vi "update facade.vi"(0 "control ref":refnum<vi>, 2 "Data In":T1, 4 "index":i32) -> (19 "error out":errorcluster)   [LabVIEW 2014, in "X DIM conditions.xctl"]
uses:
  X DIM conditions.xctl
  X DIM conditions.Data.ctl
  PTSequencer/PTSequencer.DIM service condition.ctl
  CS_Core/CSSystem/CoreDefs/CoreDefs.rawDataType.ctl
  PTSequencer/PTSequencer.lvlib
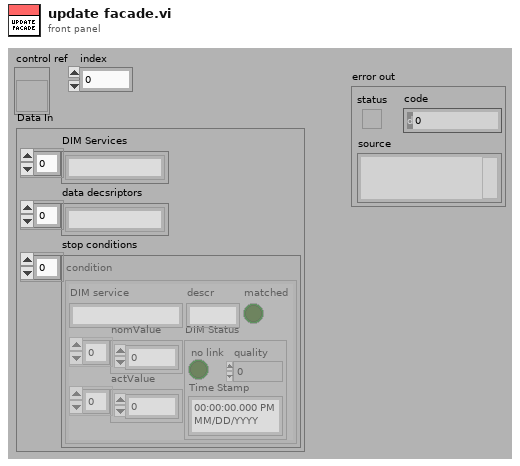
[diagram p1: front panel]
types:
  T1 = typedef "X DIM conditions.xctl/X DIM conditions.Data.ctl" = cluster{"DIM Services":string[], "data decsriptors":string[], "stop conditions":T2[]}
  T2 = typedef "PTSequencer.lvlib/PTSequencer.DIM service condition.ctl" = cluster{"DIM service":string, "descr":string, "nomValue":T3, "actValue":T3, "matched":bool, "DIM Status":cluster{"no link":bool, "quality":i32, "Time Stamp":timestamp}}
  T3 = typedef "CoreDefs.rawDataType.ctl" = i8[]
  T4 = enum8{"Enabled", "Disabled", "Disabled and Grayed Out"}
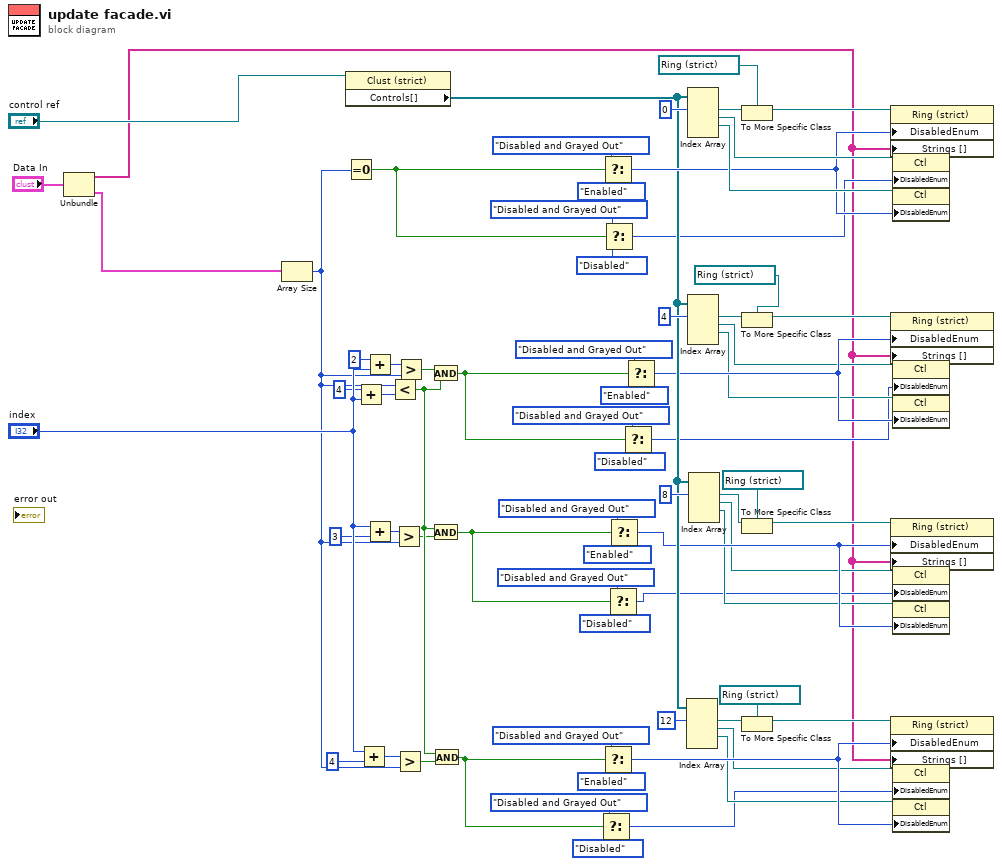
[diagram p0: block diagram]
diagram:
  n1 = Unbundle("Data In") -> ("DIM Services"=w1:string[], "stop conditions"=w69:T2[])  [unwired: 1 out]
  n2 = Array Size(array=w69) -> (size(s)=w43:i32)
  n3 = property class="Clust (strict)"(reference="control ref") -> ("Controls[]"=w39:refnum<vi>[])  [unwired: 1 in, 2 out]
  n4 = Equal To 0?(x=w43) -> (x = 0?=w6:bool)
  n5 = Add(x=4, y="index") -> (x+y=w52:i32)
  n6 = Add(x="index", y=4) -> (x+y=w56:i32)
  n7 = Add(x=2, y="index") -> (x+y=w53:i32)
  n8 = Add(x="index", y=3) -> (x+y=w55:i32)
  n9 = Less?(x=w43, y=w52) -> (x < y?=w50:bool)
  n10 = Greater?(x=w55, y=w43) -> (0:w48:bool)
  n11 = Greater?(x=w56, y=w43) -> (0:w49:bool)
  n12 = Greater?(x=w53, y=w43) -> (0:w47:bool)
  n13 = And(x=w47, y=w50) -> (x .and. y?=w7:bool)
  n14 = And(x=w50, y=w48) -> (x .and. y?=w5:bool)
  n15 = And(x=w50, y=w49) -> (x .and. y?=w8:bool)
  n16 = Select(t=T4."Disabled and Grayed Out" ("Disabled"), s=w8, f=T4."Disabled" ("Disabled")) -> (s? t:f=w12:T4)
  n17 = Select(t=T4."Disabled and Grayed Out" ("Disabled"), s=w6, f=T4."Enabled" ("Disabled")) -> (s? t:f=w40:T4)
  n18 = Select(t=T4."Disabled and Grayed Out" ("Disabled"), s=w8, f=T4."Enabled" ("Disabled")) -> (s? t:f=w27:T4)
  n19 = Select(t=T4."Disabled and Grayed Out" ("Disabled"), s=w6, f=T4."Disabled" ("Disabled")) -> (s? t:f=w11:T4)
  n20 = Select(t=T4."Disabled and Grayed Out" ("Disabled"), s=w5, f=T4."Disabled" ("Disabled")) -> (s? t:f=w13:T4)
  n21 = Select(t=T4."Disabled and Grayed Out" ("Disabled"), s=w5, f=T4."Enabled" ("Disabled")) -> (s? t:f=w28:T4)
  n22 = Select(t=T4."Disabled and Grayed Out" ("Disabled"), s=w7, f=T4."Disabled" ("Disabled")) -> (s? t:f=w14:T4)
  n23 = Select(t=T4."Disabled and Grayed Out" ("Disabled"), s=w7, f=T4."Enabled" ("Disabled")) -> (s? t:f=w33:T4)
  n24 = Index Array(array=w39, index #1=12) -> (element #1=w34:refnum<vi>, element #2=w22:refnum<vi>, element #3=w21:refnum<vi>)  [unwired: 3 in, 1 out]
  n25 = Index Array(array=w39, index #1=0) -> (element #1=w62:refnum<vi>, element #2=w60:refnum<vi>, element #3=w59:refnum<vi>)  [unwired: 3 in, 1 out]
  n26 = Index Array(array=w39, index #1=4) -> (element #1=w36:refnum<vi>, element #2=w26:refnum<vi>, element #3=w25:refnum<vi>)  [unwired: 3 in, 1 out]
  n27 = Index Array(array=w39, index #1=8) -> (element #1=w35:refnum<vi>, element #2=w24:refnum<vi>, element #3=w23:refnum<vi>)  [unwired: 3 in, 1 out]
  n28 = To More Specific Class(target class=refnum<vi> refnum ("Name 1"), reference=w62) -> (specific class reference=w63:refnum<vi>)  [unwired: 1 in, 1 out]
  n29 = To More Specific Class(target class=refnum<vi> refnum ("Name 1"), reference=w36) -> (specific class reference=w64:refnum<vi>)  [unwired: 1 in, 1 out]
  n30 = To More Specific Class(target class=refnum<vi> refnum ("Name 1"), reference=w35) -> (specific class reference=w65:refnum<vi>)  [unwired: 1 in, 1 out]
  n31 = To More Specific Class(target class=refnum<vi> refnum ("Name 1"), reference=w34) -> (specific class reference=w66:refnum<vi>)  [unwired: 1 in, 1 out]
  n32 = property class="Ring (strict)"(reference=w63, "DisabledEnum"=w40, "Strings []"=w1) -> ()  [unwired: 1 in, 2 out]
  n33 = property class="Ring (strict)"(reference=w64, "DisabledEnum"=w33, "Strings []"=w1) -> ()  [unwired: 1 in, 2 out]
  n34 = property class="Ring (strict)"(reference=w65, "DisabledEnum"=w28, "Strings []"=w1) -> ()  [unwired: 1 in, 2 out]
  n35 = property class="Ring (strict)"(reference=w66, "DisabledEnum"=w27, "Strings []"=w1) -> ()  [unwired: 1 in, 2 out]
  n36 = property class="Ctl"(reference=w60, "DisabledEnum"=w11) -> ()  [unwired: 1 in, 2 out]
  n37 = property class="Ctl"(reference=w59, "DisabledEnum"=w40) -> ()  [unwired: 1 in, 2 out]
  n38 = property class="Ctl"(reference=w26, "DisabledEnum"=w14) -> ()  [unwired: 1 in, 2 out]
  n39 = property class="Ctl"(reference=w25, "DisabledEnum"=w33) -> ()  [unwired: 1 in, 2 out]
  n40 = property class="Ctl"(reference=w24, "DisabledEnum"=w13) -> ()  [unwired: 1 in, 2 out]
  n41 = property class="Ctl"(reference=w23, "DisabledEnum"=w28) -> ()  [unwired: 1 in, 2 out]
  n42 = property class="Ctl"(reference=w22, "DisabledEnum"=w12) -> ()  [unwired: 1 in, 2 out]
  n43 = property class="Ctl"(reference=w21, "DisabledEnum"=w27) -> ()  [unwired: 1 in, 2 out]
